vi "SubVI_Izhikevich_BasicModel_005.vi"(3 "u(t)":dbl, 4 "v(0)":dbl, 5 "I":dbl(slide) scale=0.0..10.0, 6 "Model parameters":cluster{"a":dbl, "b":dbl, "c":dbl, "d":dbl}) -> (0 "u(t+dt)":dbl, 1 "v(t+dt)":dbl, 2 "Spike?":bool)   [LabVIEW 2018]
panel:
  out "u":dbl(graph)
  out "v(t+dt)":dbl(graph)
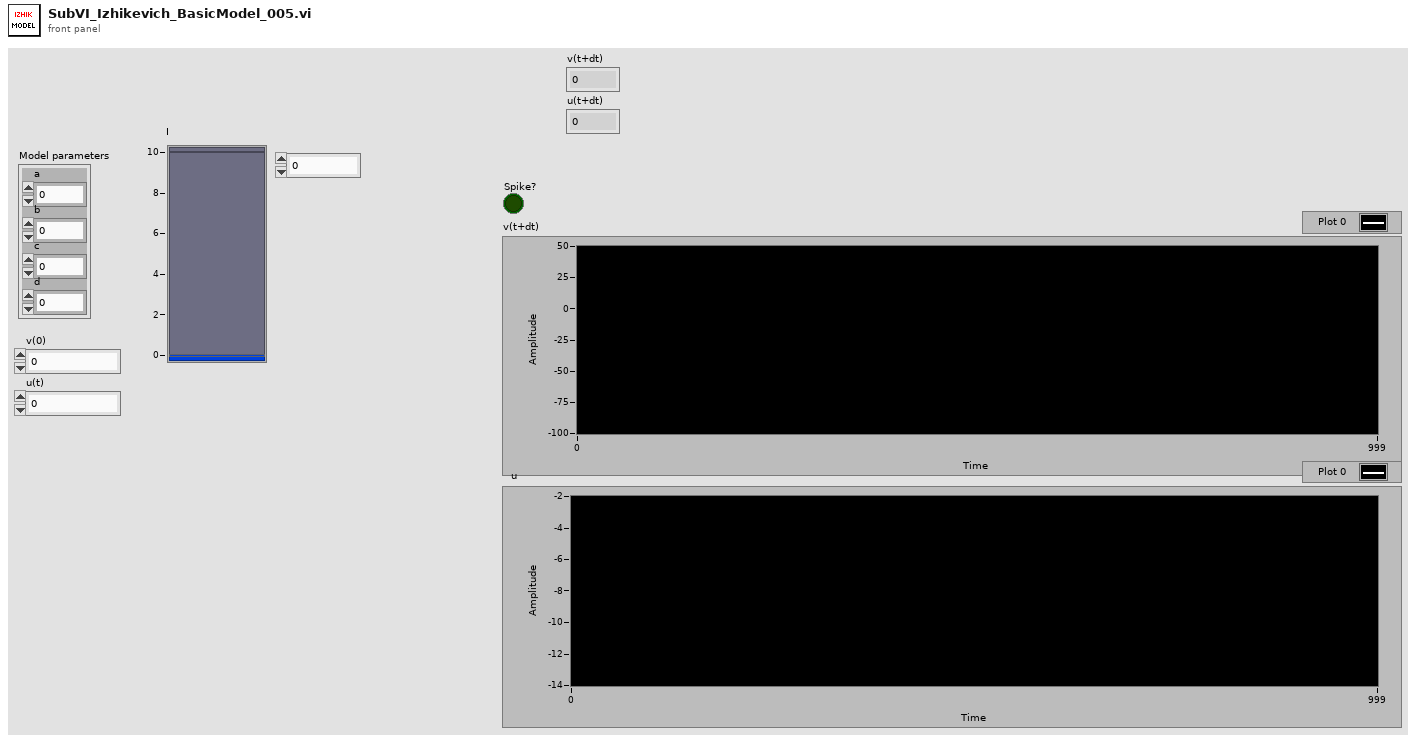
[diagram p1: front panel]
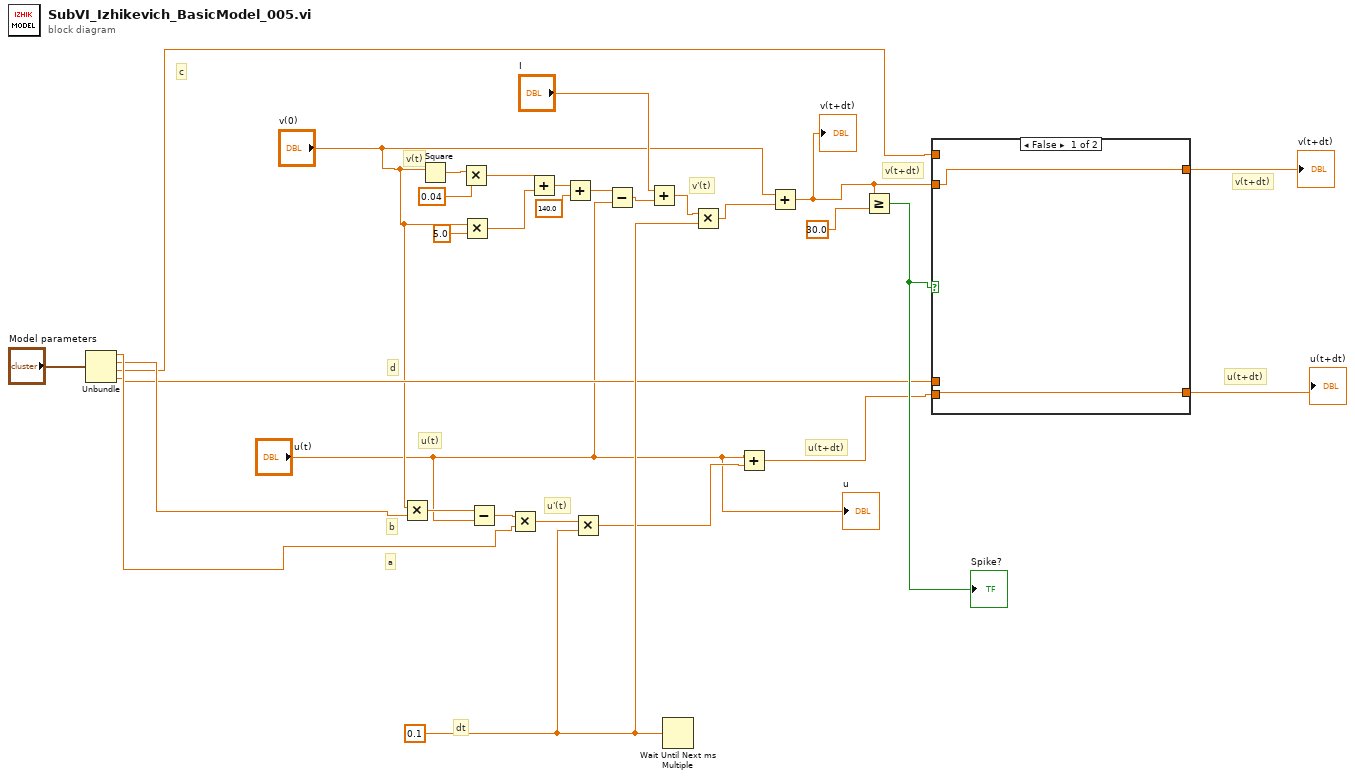
[diagram p0: block diagram]
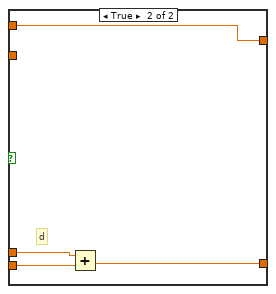
[diagram p2: hidden frame]
diagram:
  w15 = 0.1 ("millisecond multiple")
  # "u(t+dt)"
  # "c"
  # "d"
  # "b"
  # "a"
  # "u(t+dt)"
  # "v(t+dt)"
  # "u'(t)"
  # "v'(t)"
  # "dt"
  # "v(t+dt)"
  # "u(t)"
  # "v(t)"
  n1 = Unbundle("Model parameters") -> ("a"=w9:dbl, "b"=w8:dbl, "c"=w7:dbl, "d"=w6:dbl)
  n2 = Multiply(x="v(0)", y=w8) -> (x*y=w18:dbl)
  n3 = Square(x="v(0)") -> (x^2=w30:dbl)
  n4 = Multiply(x=w30, y=0.04) -> (x*y=w26:dbl)
  n5 = Multiply(x="v(0)", y=5.0) -> (x*y=w27:dbl)
  n6 = Subtract(x=w18, y="u(t)") -> (x-y=w17:dbl)
  n7 = Multiply(x=w17, y=w9) -> (x*y=w16:dbl)
  n8 = Add(x=w26, y=w27) -> (x+y=w25:dbl)
  n9 = Add(x=w25, y=140.0) -> (x+y=w23:dbl)
  n10 = Multiply(x=w16, y=w15) -> (x*y=w14:dbl)
  n11 = Subtract(x=w23, y="u(t)") -> (x-y=w21:dbl)
  n12 = Add(x="I", y=w21) -> (x+y=w22:dbl)
  n13 = Wait Until Next ms Multiple(millisecond multiple=w15) -> ()  [unwired: 1 out]
  n14 = Multiply(x=w22, y=w15) -> (x*y=w19:dbl)
  n15 = Add(x="u(t)", y=w14) -> (x+y=w11:dbl)
  n16 = Add(x="v(0)", y=w19) -> (x+y=w2:dbl)
  "v(t+dt)" <- w2
  n17 = Greater Or Equal?(x=w2, y=30.0) -> (x >= y?=w12:bool)
  "Spike?" <- w12
  n18 = case shown="False" w12 {
    tunnel: w11 -> [w32 w35]
    tunnel: [w32 w34] -> w5
    tunnel: w2 -> [w31 _]
    tunnel: [w31 w36] -> w4
    tunnel: w7 -> [_ w36]
    tunnel: w6 -> [_ w33]
    frame False {
    }
    frame True {
      # "d"
      n19 = Add(x=w33, y=w35) -> (x+y=w34:dbl)
    }
  }
  "v(t+dt)" <- w4
  "u(t+dt)" <- w5
  "u" <- "u(t)"
